vi "Timing Engine.vi"(8 "Fehler (Eingang)":errorcluster, 9 "Zeitbegrenzung":dbl, 10 "Zurücksetzen":bool, 11 "Zeitfortschritt?":bool) -> (0 "Fehler (Ausgang)":errorcluster, 1 "Verstrichene Zeit":dbl, 3 "Zeit abgelaufen?":bool)   [LabVIEW 2014]
doc: "Dieses VI bestimmt bei jedem Aufruf \"dt\" (Zeitunterschied zwischen Aufrufen). Wenn der Eingang \"Zeitfortschritt?\" True ist, wird dt zur im VI gespeicherten verstrichenen Zeit hinzugefügt. Die verstrichene Zeit wird wieder auf 0 gesetzt, wenn der Eingang \"Zurücksetzen\" True ist. Der Eingang \"Zeitbegrenzung\" wird mit der verstrichenen Zeit verglichen, um festzustellen, ob die Zeit abgelaufen ist."
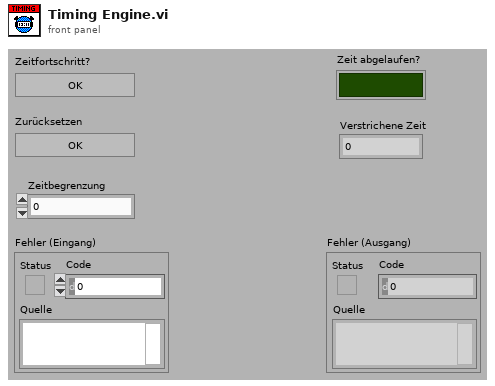
[diagram p1: front panel]
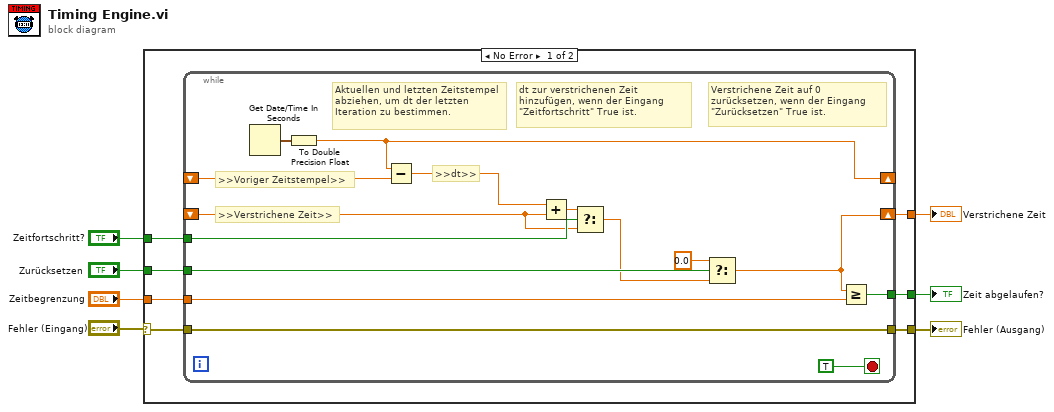
[diagram p0: block diagram]
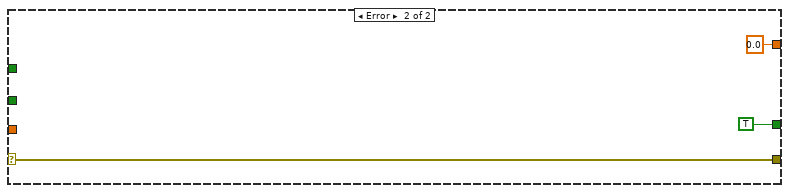
[diagram p2: hidden frame]
diagram:
  n1 = case "Case-Struktur" shown="No Error" "Fehler (Eingang)" {
    selector: "Fehler (Eingang)" -> [w8 w32]
    tunnel: "Zurücksetzen" -> [w14 _]
    tunnel: [w13 0.0 ("t")] -> w6
    tunnel: "Zeitbegrenzung" -> [w12 _]
    tunnel: [w11 TRUE] -> w4
    tunnel: "Zeitfortschritt?" -> [w10 _]
    tunnel: [w9 w32] -> w1
    frame No Error {
      n2 = while "While-Schleife" {
        shift-right: [w27] -> _
        shift-left: _ -> [w26]
        shift-right: [w22] -> w13
        shift-left: _ -> [w17]
        tunnel: w14 -> [w24]
        tunnel: w12 -> [w21]
        tunnel: [w20] -> w11
        tunnel: w10 -> [w19]
        tunnel: [w15] -> w9
        tunnel: w8 -> [w15]
        stop <- TRUE stop-if-true
        # "Verstrichene Zeit auf 0 zurücksetzen, wenn der Eingang \"Zurücksetzen\" True ist."
        # "Aktuellen und letzten Zeitstempel abziehen, um dt der letzten Iteration zu bestimmen."
        # "dt zur verstrichenen Zeit hinzufügen, wenn der Eingang \"Zeitfortschritt\" True ist."
        # ">>dt>>"
        # ">>Verstrichene Zeit>>"
        # ">>Voriger Zeitstempel>>"
        n3 = Get Date/Time In Seconds ("Datum/Zeit in Sekunden ermitteln")() -> (seconds since 1Jan1904=w28:timestamp)
        n4 = To Double Precision Float ("Nach Fließkommawert (doppelte Genauigkeit)")(number=w28) -> (double precision float=w27:dbl)
        n5 = Subtract ("Subtrahieren")(x=w27, y=w26) -> (x-y=w25:dbl)
        n6 = Add ("Addieren")(x=w25, y=w17) -> (x+y=w18:dbl)
        n7 = Select ("Auswählen")(t=w18, s=w19, f=w17) -> (s? t:f=w16:dbl)
        n8 = Select ("Auswählen")(t=0.0, s=w24, f=w16) -> (s? t:f=w22:dbl)
        n9 = Greater Or Equal? ("Größer oder gleich?")(x=w22, y=w21) -> (x >= y?=w20:bool)
      }
    }
    frame Error {
    }
  }
  "Verstrichene Zeit" <- w6
  "Zeit abgelaufen?" <- w4
  "Fehler (Ausgang)" <- w1
